vi "Transform.vi"(8 "error in (no error)":errorcluster, 11 "XRay Cabinet in":refnum<class "XRay Cabinet.lvclass">) -> (0 "error out":errorcluster, 3 "XRay Cabinet out":refnum<class "XRay Cabinet.lvclass">)   [LabVIEW 2026, in "XRay Cabinet.lvclass"]
uses:
  XRay Cabinet.lvclass
  XRay Cabinet.lvclass/XRay Cabinet.ctl
  XRay Scene/XRay Scene.lvclass
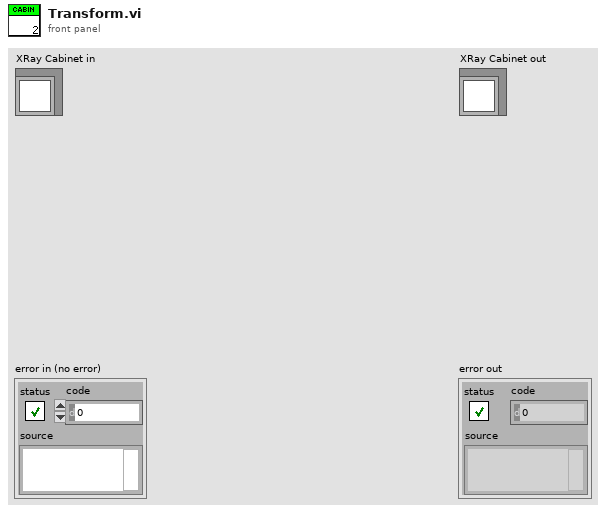
[diagram p1: front panel]
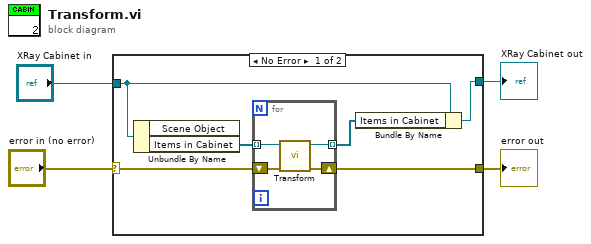
[diagram p0: block diagram]
diagram:
  n1 = case shown="No Error" "error in (no error)" {
    selector: "error in (no error)" -> [w6 w16]
    tunnel: [w5 w16] -> w3
    tunnel: [w7 w15] -> w1
    tunnel: "XRay Cabinet in" -> [w8 w15]
    frame No Error {
      n2 = Unbundle By Name(w8) -> ("Items in Cabinet"=w10:refnum<class "XRay Scene.lvclass">[])  [unwired: 1 out]
      n3 = for {
        tunnel: w10 -> [w14] mode=indexing
        tunnel: [w13] -> w9 mode=indexing
        shift-right: [w11] -> w5
        shift-left: w6 -> [w12]
        n4 = call-dynamic "Transform.vi"("error in (no error)"=w12, "XRay Scene in"=w14) -> ("error out"=w11:errorcluster, "XRay Scene out"=w13:refnum<class "XRay Scene.lvclass">)  [unwired: 8 in]
      }
      n5 = Bundle By Name(cluster=w8, "Items in Cabinet"=w9) -> (w7:refnum<class "XRay Cabinet.lvclass">)
    }
    frame Error {
    }
  }
  "error out" <- w3
  "XRay Cabinet out" <- w1
